vi "Override Null objects.vi"(8 "error in (no error)":errorcluster, 9 "Columns":refnum<class "GridColumn.lvclass">[](array[class]), 11 ".NET Refnum in":refnum<k24>) -> (0 "error out":errorcluster)   [LabVIEW 2016, in "DataGrid.lvlib" / "DataGridView.lvclass"]
doc: "Defines the null value types for buttons and images, so they can be empty strings, without breaking the data types for those columns."
uses:
  <userlib>/LabVIEWdotNetDataGrid/source/DataGridView/DataGridView.lvclass
  System.Windows.Forms
  <userlib>/LabVIEWdotNetDataGrid/source/GridColumn/GridColumn.lvclass
  <userlib>/LabVIEWdotNetDataGrid/source/GridColumn/GridColumn.lvclass/GridColumn.ctl
  <userlib>/LabVIEWdotNetDataGrid/source/GridColumn/Read datatype.vi
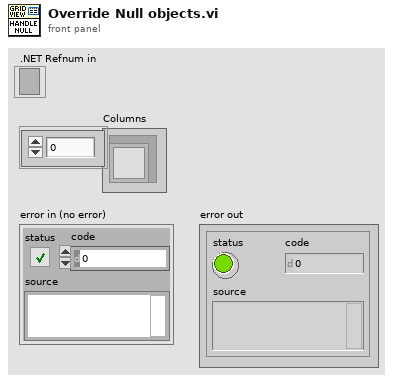
[diagram p1: front panel]
types:
  T1 = typedef "DataGrid.lvlib/GridColumn.lvclass/ColumnType.ctl" = enum16{"string", "image", "check", "numeric", "timestamp", "button", "combo", "link"}
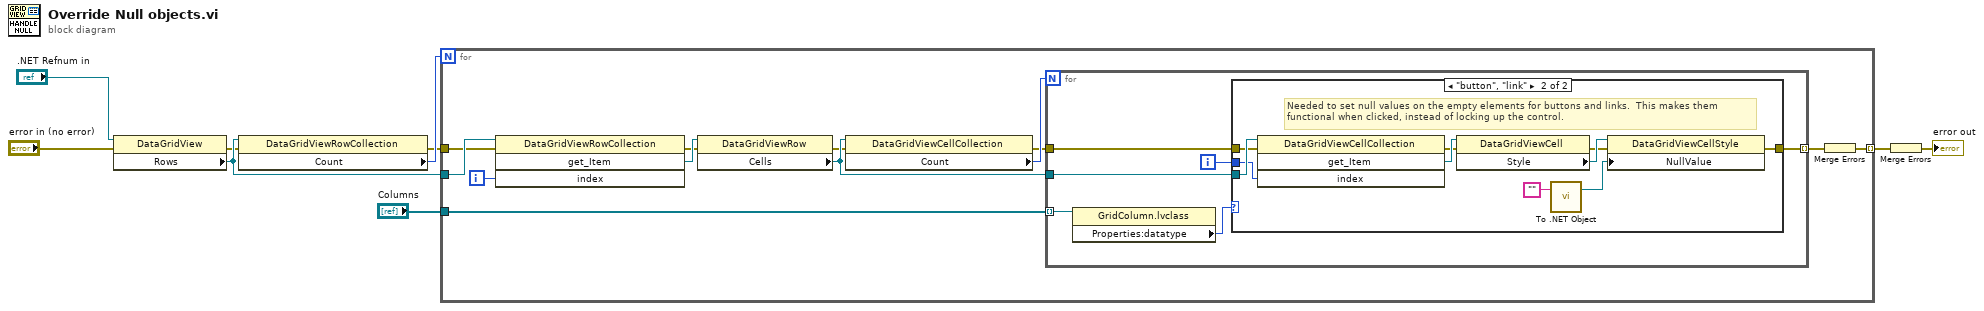
[diagram p0: block diagram]
diagram:
  n1 = property class="DataGridView"(reference=".NET Refnum in", error in="error in (no error)") -> (error out=w6:errorcluster, "Rows"=w8:refnum<k24>)  [unwired: 1 out]
  n2 = property class="DataGridViewRowCollection"(reference=w8, error in=w6) -> (error out=w5:errorcluster, "Count"=w7:i32)  [unwired: 1 out]
  n3 = for {
    N: w7 -> [_]
    tunnel: w8 -> [w21]
    tunnel: w5 -> [w16]
    tunnel: [w11] -> w4 mode=indexing
    tunnel: "Columns" -> [w10]
    i -> [w20]
    n4 = invoke class="DataGridViewRowCollection" method="get_Item"(reference=w21, error in=w16, "index"=w20) -> (error out=w15:errorcluster, "get_Item"=w19:refnum<k24>)  [unwired: 1 in, 2 out]
    n5 = property class="DataGridViewRow"(reference=w19, error in=w15) -> (error out=w14:errorcluster, "Cells"=w18:refnum<k24>)  [unwired: 1 out]
    n6 = property class="DataGridViewCellCollection"(reference=w18, error in=w14) -> (error out=w13:errorcluster, "Count"=w17:i32)  [unwired: 1 out]
    n7 = for {
      N: w17 -> [_]
      tunnel: w18 -> [w27]
      tunnel: w13 -> [w25]
      tunnel: [w24] -> w12 mode=indexing
      tunnel: w10 -> [w23] mode=indexing
      i -> [w26]
      n8 = property class="GridColumn.lvclass"(reference=w23) -> ("Properties:datatype"=w22:T1)  [unwired: 1 in, 2 out]
      n9 = case shown="\"button\", \"link\"" w22 {
        tunnel: w27 -> [_ w38]
        tunnel: w26 -> [_ w37]
        tunnel: w25 -> [w28 w36]
        tunnel: [w28 w31] -> w24
        frame Default {
        }
        frame "button", "link" {
          # "Needed to set null values on the empty elements for buttons and links.  This makes them\nfunctional when clicked, instead of locking up the control."
          n10 = invoke class="DataGridViewCellCollection" method="get_Item"(reference=w38, error in=w36, "index"=w37) -> (error out=w33:errorcluster, "get_Item"=w35:refnum<k24>)  [unwired: 1 in, 2 out]
          n11 = property class="DataGridViewCell"(reference=w35, error in=w33) -> (error out=w32:errorcluster, "Style"=w34:refnum<k24>)  [unwired: 1 out]
          n12 = call <vilib>:"To .NET Object.vi"("anything"="") -> (".NET object"=w29:refnum<k24>)  [unwired: 1 in, 1 out]
          n13 = property class="DataGridViewCellStyle"(reference=w34, error in=w32, "NullValue"=w29) -> (error out=w31:errorcluster)  [unwired: 1 out]
        }
      }
    }
    n14 = Merge Errors(w12) -> (w11:errorcluster)
  }
  n15 = Merge Errors(w4) -> (→"error out":errorcluster)
